vi "snap_qrcode_numpy.vi"() -> ()   [LabVIEW 2018]
panel:
  out "Input QR Code":picture
  out "Output QR Code":picture
  out "return value":cluster{"found":i32, "decode data":string}
  in  "Output image filename":string="decode.png"
  in  "QR Code Image Path":path=path "hello.png"
  # "Free QR code generator website"
  # "https://www.the-qrcode-generator.com/"
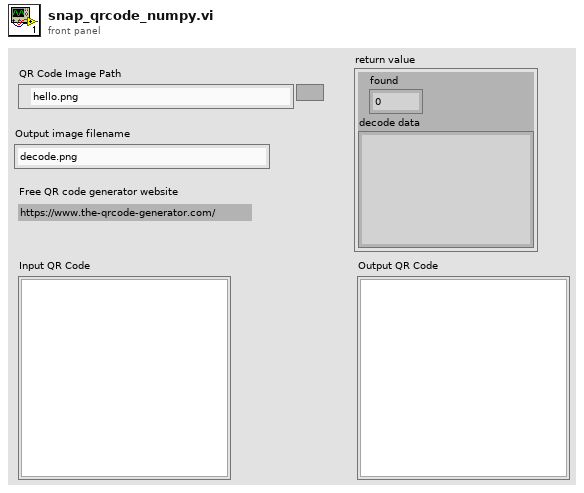
[diagram p1: front panel]
types:
  T1 = typedef "imagedata.ctl" = cluster{"image type":i32, "image depth":i32, "image":u8[], "mask":u8[], "colors":u32[], "Rectangle":cluster{"left":i16, "top":i16, "right":i16, "bottom":i16}}
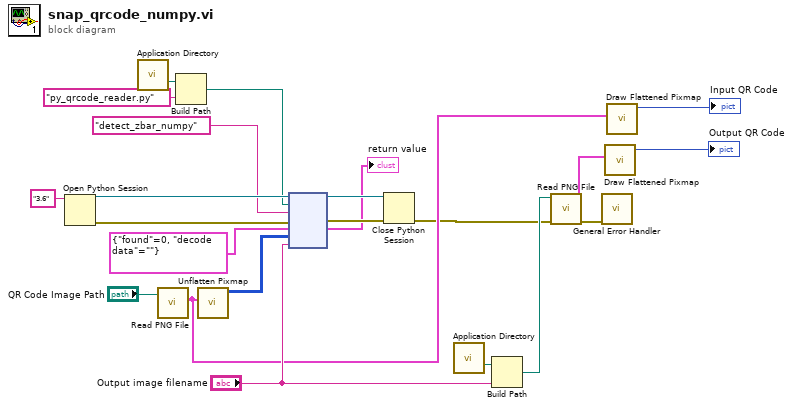
[diagram p0: block diagram]
diagram:
  n1 = Open Python Session(python version="3.6" ("Python version")) -> (session out=w21:refnum<k35>, error out=w19:errorcluster)  [unwired: 2 in]
  n2 = call <vilib>:"Application Directory.vi"() -> ("Application Directory"=w11:path)
  n3 = call <vilib>:"Read PNG File.vi"("path to PNG file"="QR Code Image Path") -> ("image data"=w2:T1)  [unwired: 8 in, 2 out]
  n4 = Build Path(base path=w11, name or relative path="py_qrcode_reader.py" ("module filename")) -> (appended path=w9:path)
  n5 = call <vilib>:"Unflatten Pixmap.vi"("image data"=w2) -> ("24-bit pixmap"=w3:u32[][])  [unwired: 4 in, 6 out]
  n6 = node(w21, w9, "detect_zbar_numpy" ("function name"), w19, cluster{"found":i32, "decode data":string} {"found"=0, "decode data"=""}, w3, "Output image filename") -> (w20:refnum<k35>, w18:errorcluster, →"return value":cluster{"found":i32, "decode data":string})  [unwired: 2 in, 2 out]
  n7 = Close Python Session(session in=w20, error in=w18) -> (11:w1:errorcluster)
  n8 = call <vilib>:"Application Directory.vi"() -> ("Application Directory"=w16:path)
  n9 = Build Path(base path=w16, name or relative path="Output image filename") -> (appended path=w15:path)
  n10 = call <vilib>:"Read PNG File.vi"("error in (no error)"=w1, "path to PNG file"=w15) -> ("error out"=w12:errorcluster, "image data"=w14:T1)  [unwired: 7 in, 1 out]
  n11 = call <vilib>:"General Error Handler.vi"("error in (no error)"=w12) -> ()  [unwired: 10 in, 5 out]
  n12 = call <vilib>:"Draw Flattened Pixmap.vi"("image data"=w14) -> ("new picture"=→"Output QR Code":picture)  [unwired: 8 in]
  n13 = call <vilib>:"Draw Flattened Pixmap.vi"("image data"=w2) -> ("new picture"=→"Input QR Code":picture)  [unwired: 8 in]
